vi "Get Authority.vi"(8 "error in (no error)":errorcluster, 11 "URI in":refnum<class "URI.lvclass">) -> (0 "error out":errorcluster, 2 "Authority":string, 3 "URI out":refnum<class "URI.lvclass">)   [LabVIEW 2020, in "Stream.lvlib" / "URI.lvclass"]
uses:
  URI.lvclass
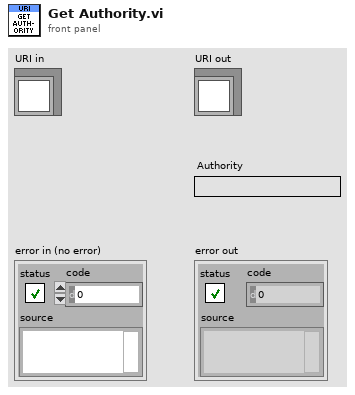
[diagram p1: front panel]
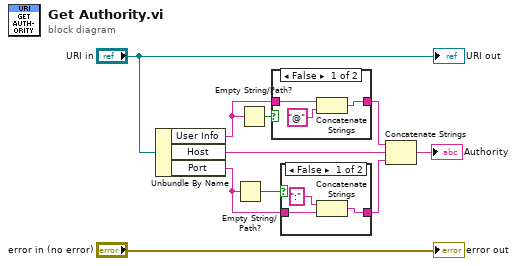
[diagram p0: block diagram]
diagram:
  n1 = Unbundle By Name("URI in") -> ("User Info"=w5:string, "Host"=w4:string, "Port"=w7:string)
  n2 = Empty String/Path?(string/path=w7) -> (empty?=w8:bool)
  n3 = Empty String/Path?(string/path=w5) -> (empty?=w6:bool)
  n4 = case shown="False" w6 {
    tunnel: w5 -> [w13 w14]
    tunnel: [w12 w14] -> w3
    frame False {
      n5 = Concatenate Strings(w13, "@" ("string")) -> (w12:string)
    }
    frame True {
    }
  }
  n6 = case shown="False" w8 {
    tunnel: w7 -> [w17 w18]
    tunnel: [w15 w18] -> w2
    frame False {
      n7 = Concatenate Strings(":" ("string"), w17) -> (w15:string)
    }
    frame True {
    }
  }
  n8 = Concatenate Strings(w3, w4, w2) -> (→"Authority":string)
  "error out" <- "error in (no error)"
  "URI out" <- "URI in"
